vi "test bdd.vi"() -> ()   [LabVIEW 2020]
panel:
  in  "SEND":bool
  out "errout":errorcluster
  in  "errin":errorcluster
  in  "INSERT":string
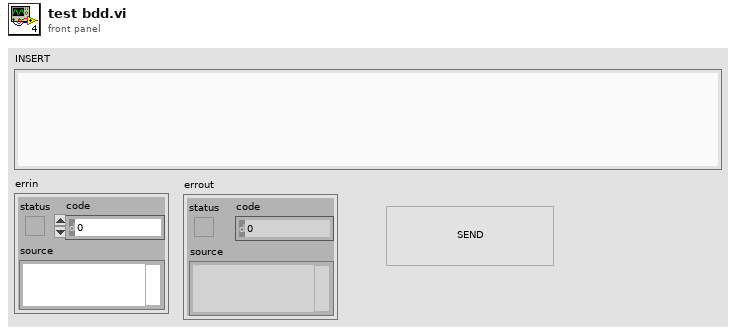
[diagram p1: front panel]
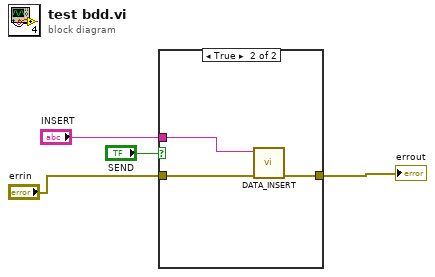
[diagram p0: block diagram]
diagram:
  n1 = case shown="True" "SEND" {
    tunnel: "INSERT" -> [_ w8]
    tunnel: [w5 w7] -> w3
    tunnel: "errin" -> [w5 w6]
    frame False {
    }
    frame True {
      n2 = call <userlib>:"DATA_INSERT.vi"("errin"=w6, "INSERT"=w8) -> ("errout"=w7:errorcluster)  [unwired: 9 in]
    }
  }
  "errout" <- w3
